vi "G#Object_QualifiedNameArrayToSingleString.vi"(1 "Fully Qualified Array":string[](array[string])) -> (0 "Fully Qualified String":string)   [LabVIEW 2017, in "G#Object.lvclass"]
doc: "The fully qualified name of a LabVIEW file is the names of all libraries that own the file followed by the name of the file itself. So if Alpha.VI is owned by a LabVIEW class X.lvclass and the class is itself owned by a library Q.lvlib, then the fully qualified name of the VI is \"Q.lvlib:X.lvclass:Alpha.vi\". Frequently qualified names on the block diagram are handled as arrays of strings, useful when displaying the name in some tree structure. This function translates an array of strings into a single string using the colon as a delimiter, which is how the name is displayed inline, such as the VI's window title."
uses:
  G#Object.lvclass
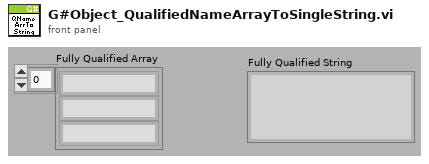
[diagram p1: front panel]
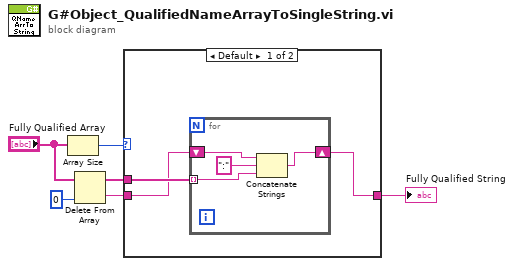
[diagram p0: block diagram]
diagram:
  n1 = Array Size(array="Fully Qualified Array") -> (size(s)=w6:i32)
  n2 = Delete From Array(array="Fully Qualified Array", index=0) -> (deleted portion=w3:string, array with subset deleted=w2:string[])  [unwired: 1 in]
  n3 = case shown="Default" w6 {
    tunnel: w3 -> [w8 w14]
    tunnel: w2 -> [w9 _]
    tunnel: [w7 w14] -> w1
    frame Default {
      n4 = for {
        tunnel: w9 -> [w11] mode=indexing
        shift-right: [w10] -> w7
        shift-left: w8 -> [w12]
        n5 = Concatenate Strings(w12, ":" ("string"), w11) -> (w10:string)
      }
    }
    frame 0, 1 {
    }
  }
  "Fully Qualified String" <- w1
